vi "Untitled 2.vi"() -> ()   [LabVIEW 2013]
uses:
  <vilib>/Rock Robotics/WPI/Relay/WPI_RelayValue.ctl
panel:
  in  "Bottom limit switch":bool
  in  "Top limit switch":bool
  in  "Botton on":bool
  in  "stop":bool
  out "Blocker State":T1
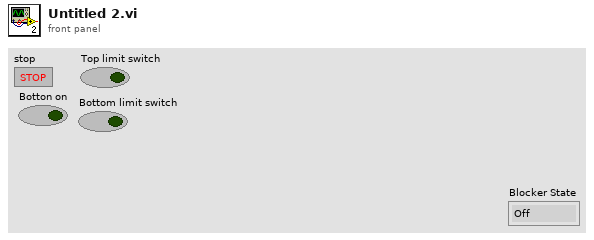
[diagram p1: front panel]
types:
  T1 = typedef "WPI_RelayValue.ctl" = enum16{"Off", "On", "Forward", "Reverse"}
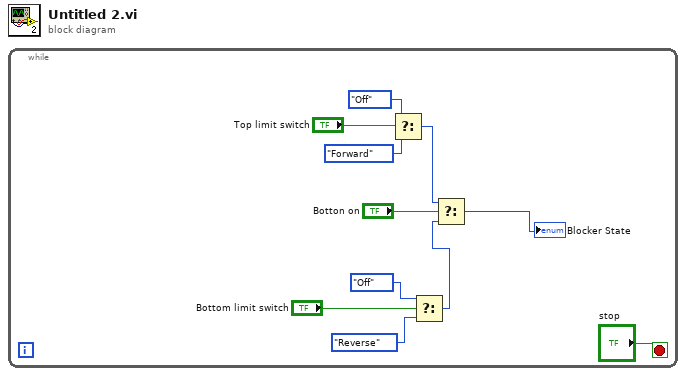
[diagram p0: block diagram]
diagram:
  n1 = while {
    stop <- "stop" stop-if-true
    n2 = Select(t=WPI_RelayValue."Off" ("Blocker State"), s="Top limit switch", f=WPI_RelayValue."Forward" ("Blocker State")) -> (s? t:f=w6:T1)
    n3 = Select(t=WPI_RelayValue."Off" ("Blocker State"), s="Bottom limit switch", f=WPI_RelayValue."Reverse" ("Blocker State")) -> (s? t:f=w3:T1)
    n4 = Select(t=w6, s="Botton on", f=w3) -> (s? t:f=→"Blocker State":T1)
  }
